vi "Get Motor Status.vi"(8 "error in (no error)":errorcluster, 11 "SDO object in":refnum<k20>) -> (0 "error out":errorcluster, 2 "Motor Status":T1, 3 "SDO object out":refnum<k20>)   [LabVIEW 2016]
uses:
  Get Statusword.vi
  Get Controller Temperature.vi
  Get Motor Temperature.vi
  Get Error.vi
  Get Error Register.vi
  Get Torque Actual Value.vi
  Get Velocity Actual Value.vi
  Get Electrical Angle.vi
  Get Electric Power.vi
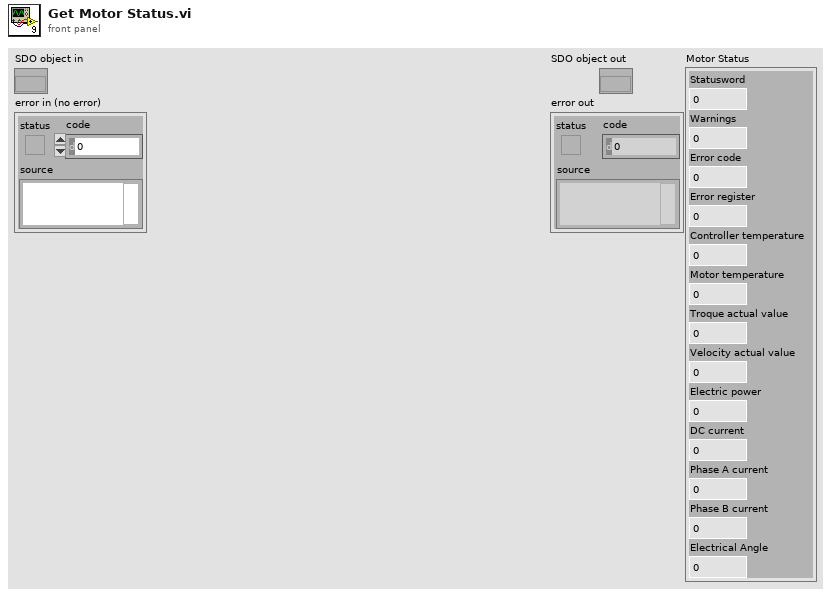
[diagram p1: front panel]
types:
  T1 = cluster{"Statusword":u16, "Warnings":u16, "Error code":u16, "Error register":u8, "Controller temperature":u8, "Motor temperature":u8, "Troque actual value":i16, "Velocity actual value":i32, "Electric power":u32, "DC current":u32, "Phase A current":u16, "Phase B current":u16, "Electrical Angle":u16}
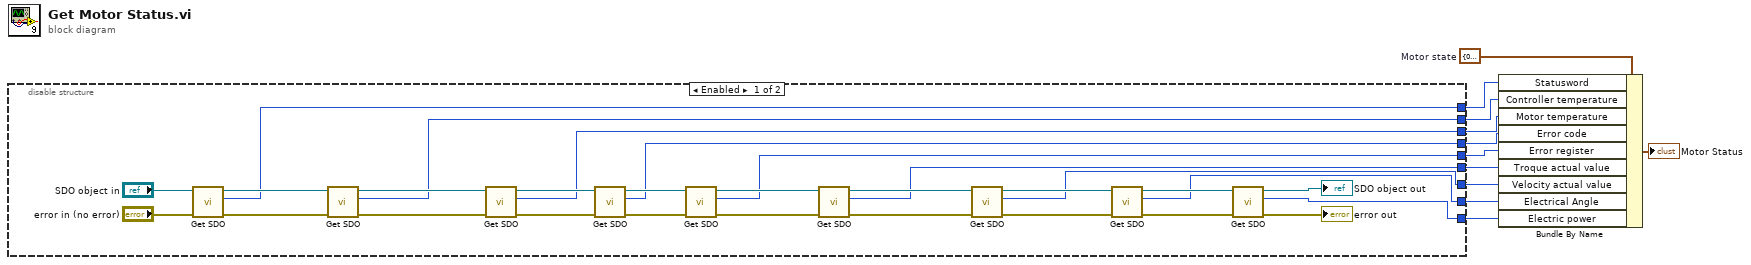
[diagram p0: block diagram]
diagram:
  w11 = T1 {"Statusword"=0, "Warnings"=0, "Error code"=0, "Error register"=0, "Controller temperature"=0, "Motor temperature"=0, "Troque actual value"=0, "Velocity actual value"=0, "Electric power"=0, "DC current"=0, "Phase A current"=0, "Phase B current"=0, "Electrical Angle"=0}  # Motor state
  n1 = disable-structure shown="Enabled" {
    disable-tunnel: [w20 _] -> w10
    disable-tunnel: [w19 _] -> w9
    disable-tunnel: [w18 _] -> w8
    disable-tunnel: [w17 _] -> w7
    disable-tunnel: [w16 _] -> w6
    disable-tunnel: [w15 _] -> w5
    disable-tunnel: [w14 _] -> w4
    disable-tunnel: [w13 _] -> w3
    disable-tunnel: [w12 _] -> w2
    frame Enabled {
      n2 = call-poly "Get SDO.vi"("error in (no error)"="error in (no error)", "SDO object in"="SDO object in") -> ("error out"=w28:errorcluster, "Status word"=w20:u16, "SDO object out"=w39:refnum<k20>)  [unwired: 6 in, 1 out]
      n3 = call-poly "Get SDO.vi"("error in (no error)"=w28, "SDO object in"=w39) -> ("error out"=w27:errorcluster, "U8 data"=w19:u8, "SDO object out"=w38:refnum<k20>)  [unwired: 6 in, 1 out]
      n4 = call-poly "Get SDO.vi"("error in (no error)"=w27, "SDO object in"=w38) -> ("error out"=w26:errorcluster, "U8 data"=w18:u8, "SDO object out"=w37:refnum<k20>)  [unwired: 6 in, 1 out]
      n5 = call-poly "Get SDO.vi"("error in (no error)"=w26, "SDO object in"=w37) -> ("error out"=w25:errorcluster, "Error code"=w17:u16, "SDO object out"=w36:refnum<k20>)  [unwired: 5 in, 2 out]
      n6 = call-poly "Get SDO.vi"("error in (no error)"=w25, "SDO object in"=w36) -> ("error out"=w24:errorcluster, "U8 data"=w16:u8, "SDO object out"=w35:refnum<k20>)  [unwired: 6 in, 1 out]
      n7 = call-poly "Get SDO.vi"("error in (no error)"=w24, "SDO object in"=w35) -> ("error out"=w23:errorcluster, "I32 data"=w15:i16, "SDO object out"=w34:refnum<k20>)  [unwired: 6 in, 1 out]
      n8 = call-poly "Get SDO.vi"("error in (no error)"=w23, "SDO object in"=w34) -> ("error out"=w22:errorcluster, "I32 data"=w14:i32, "SDO object out"=w33:refnum<k20>)  [unwired: 6 in, 1 out]
      n9 = call-poly "Get SDO.vi"("error in (no error)"=w22, "SDO object in"=w33) -> ("error out"=w21:errorcluster, "I32 data"=w12:i16, "SDO object out"=w32:refnum<k20>)  [unwired: 6 in, 1 out]
      n10 = call-poly "Get SDO.vi"("error in (no error)"=w21, "SDO object in"=w32) -> ("error out"=→"error out":errorcluster, "I32 data"=w13:u32, "SDO object out"=→"SDO object out":refnum<k20>)  [unwired: 6 in, 1 out]
    }
    frame Disabled {
    }
  }
  n11 = Bundle By Name(cluster=w11, "Statusword"=w10, "Controller temperature"=w9, "Motor temperature"=w8, "Error code"=w7, "Error register"=w6, "Troque actual value"=w5, "Velocity actual value"=w4, "Electrical Angle"=w2, "Electric power"=w3) -> (→"Motor Status":T1)
